vi "ConfigFileDialog.vi"(8 "Error In":errorcluster, 10 "folder name":string, 11 "Path":path) -> (0 "Error Out":errorcluster, 2 "cancelled dialog?":bool caption="cancelled", 3 "Output path":path caption="selected path")   [LabVIEW 2014]
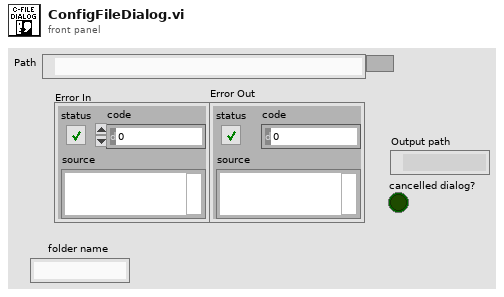
[diagram p1: front panel]
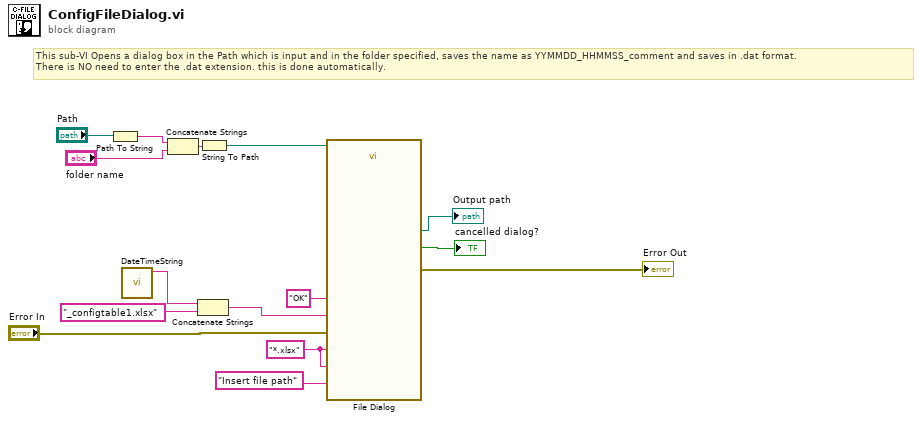
[diagram p0: block diagram]
diagram:
  w1 = "*.xlsx" ("pattern (all files)")
  # "This sub-VI Opens a dialog box in the Path which is input and in the folder specified, saves the name as YYMMDD_HHMMSS_comment and saves in .dat format.\nThere is NO need to enter the .dat extension. this is done automatically."
  n1 = Path To String(path="Path") -> (string=w12:string)
  n2 = call "DateTimeString.vi"() -> ("date/time string"=w9:string)  [unwired: 11 in]
  n3 = Concatenate Strings(w12, "folder name") -> (w11:string)
  n4 = Concatenate Strings(w9, "_configtable1.xlsx" ("string")) -> (w7:string)
  n5 = String To Path(string=w11) -> (path=w10:path)
  n6 = call "File Dialog"("start path"=w10, "prompt"="Insert file path", "button label"="OK", "default name"=w7, "error in"="Error In", "pattern (all files)"=w1, "pattern label"=w1) -> ("selected path"=→"Output path":path, "cancelled"=→"cancelled dialog?":bool, "error out"=→"Error Out":errorcluster)  [unwired: 5 in, 1 out]
